vi "ifr2025 Recall.vi"(8 "error in (no error)":errorcluster {"code" format="%.0x"}, 9 "Recall Number (0)":i16 format="%.0g", 10 "Recall Type (CFRQ)":i16(ring) items=["CFRQ", "FULL", "RAM", "ALL"], 11 "instrument handle":refnum<visa-resource-name>) -> (0 "error out":errorcluster {"code" format="%.0x"}, 3 "instrument handle out":refnum<visa-resource-name>)   [LabVIEW 2009]
doc: "This VI returns the instrument to the settings stored in the specified location.\n\nNote that CFRQ and FULL stores are non-volitile, but RAM contents are lost when the instrument is switched off."
uses:
  Ifr2025_32.dll
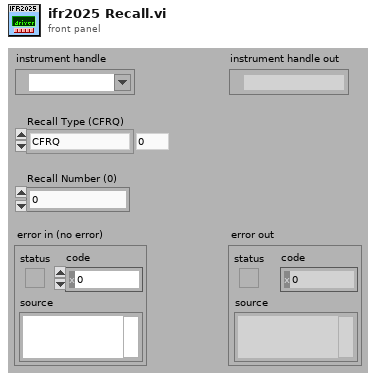
[diagram p1: front panel]
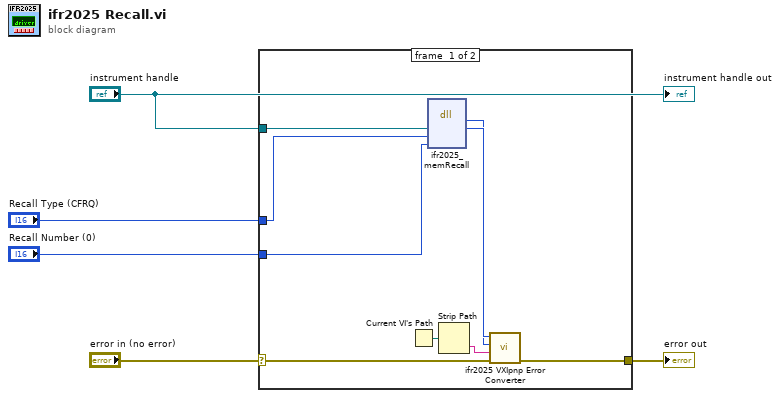
[diagram p0: block diagram]
diagram:
  n1 = case shown="No Error" "error in (no error)" {
    selector: "error in (no error)" -> [w9 w15]
    tunnel: [w8 w15] -> w5
    tunnel: "instrument handle" -> [w13 _]
    tunnel: "Recall Type (CFRQ)" -> [w7 _]
    tunnel: "Recall Number (0)" -> [w6 _]
    frame #0 {
      n2 = Current VI's Path() -> (path=w14:path)
      n3 = dll-call lib="P:/inst/Marconi 2024 Signal Generator/source/labview/ifr2025/ifr2025/ifr2025_*.*" fn="ifr2025_memRecall"("vi"=w13, "Recall Type"=w7, "Recall Number"=w6) -> (w11:i32, "vi"=w12:u32)  [unwired: 5 in, 2 out]
      n4 = Strip Path(path=w14) -> (name=w10:string)  [unwired: 1 out]
      n5 = call "ifr2025 VXIpnp Error Converter.vi"("error in (no error)"=w9, "name of VI (\"\")"=w10, "CVI error code (0)"=w11, "instrument handle"=w12) -> ("error out"=w8:errorcluster)  [unwired: 7 out]
    }
    frame #1 {
    }
  }
  "error out" <- w5
  "instrument handle out" <- "instrument handle"
